vi "_UtilsRandomI64Value.vi"(1 "factor":dbl=100.0) -> (0 "random value":i64)   [LabVIEW 2014, in "examples.lvlib"]
uses:
  examples.lvlib
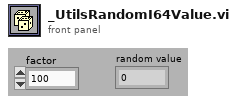
[diagram p1: front panel]
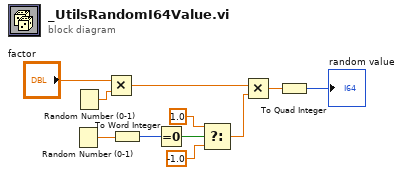
[diagram p0: block diagram]
diagram:
  n1 = Random Number (0-1)() -> (number: 0 to 1=w9:dbl)
  n2 = Random Number (0-1)() -> (number: 0 to 1=w11:dbl)
  n3 = Multiply(x="factor", y=w11) -> (x*y=w4:dbl)
  n4 = To Word Integer(number=w9) -> (16bit integer=w8:i16)
  n5 = Equal To 0?(x=w8) -> (x = 0?=w7:bool)
  n6 = Select(t=1.0 ("cas vrai"), s=w7, f=-1.0 ("cas faux")) -> (s? t:f=w3:dbl)
  n7 = Multiply(x=w4, y=w3) -> (x*y=w2:dbl)
  n8 = To Quad Integer(1:w2) -> (0:→"random value":i64)
